vi "Get name from label.vi"(8 "error in (no error)":errorcluster, 10 "Selected label":string, 11 "UI JSON read cluster":T1) -> (0 "error out":errorcluster, 3 "Diagnostic name":string)   [LabVIEW 2019, in "ZenGage v3.0 UI.lvclass"]
uses:
  ZenGage v3.0 UI.lvclass
  Type Definitions/JSON Read/UI JSON read cluster.ctl
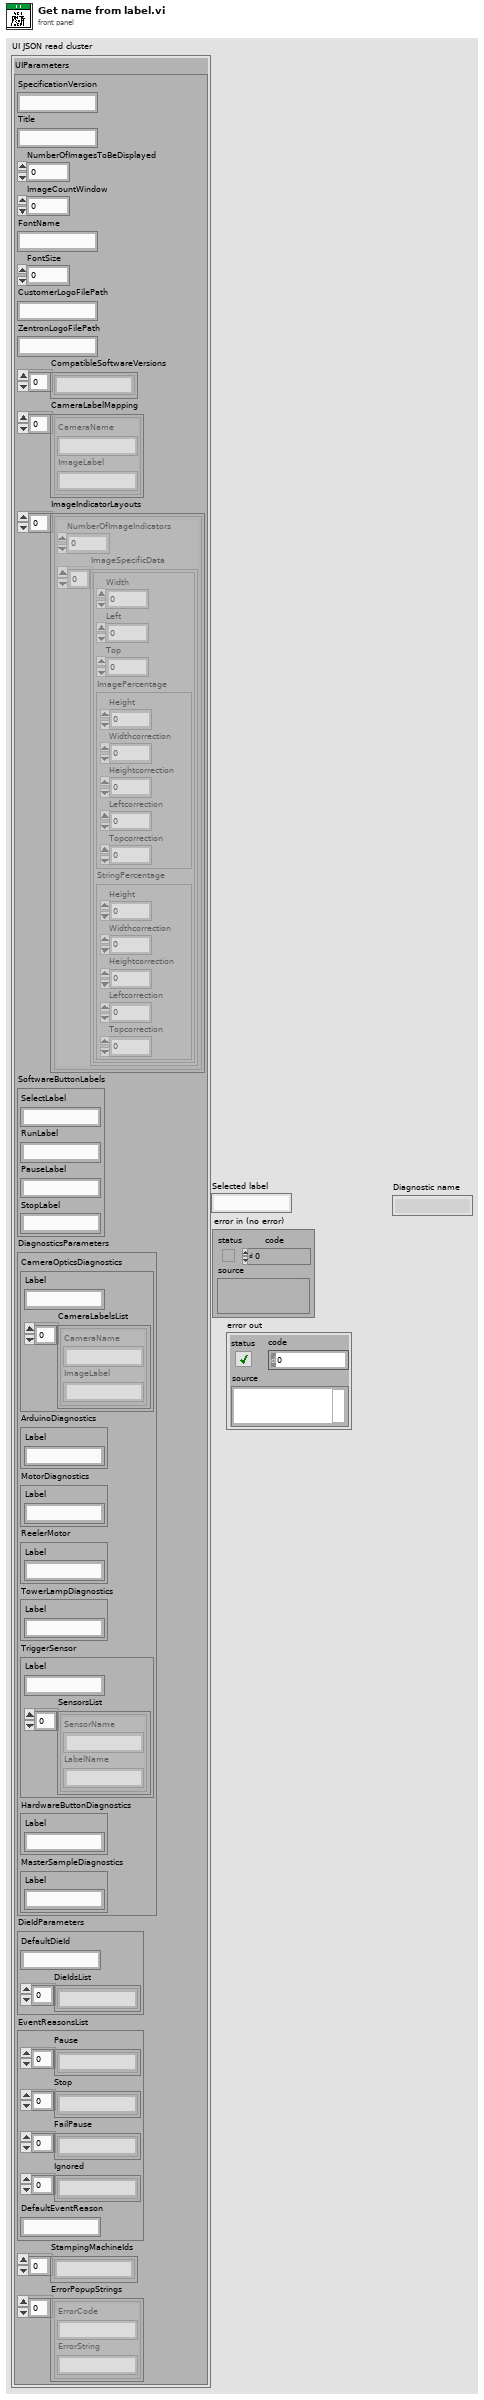
[diagram p1: front panel]
types:
  T1 = typedef "ZenGage v3.0 UI.lvclass/UI JSON read cluster.ctl" = cluster{"UIParameters":cluster{"SpecificationVersion":string, "Title":string, "NumberOfImagesToBeDisplayed":dbl, "ImageCountWindow":dbl, "FontName":string, "FontSize":dbl, "CustomerLogoFilePath":string, "ZentronLogoFilePath":string, "CompatibleSoftwareVersions":string[], "CameraLabelMapping":cluster{"CameraName":string, "ImageLabel":string}[], "ImageIndicatorLayouts":cluster{"NumberOfImageIndicators":dbl, "ImageSpecificData":cluster{"Width":dbl, "Left":dbl, "Top":dbl, "ImagePercentage":cluster{"Height":dbl, "Widthcorrection":i64, "Heightcorrection":i64, "Leftcorrection":dbl, "Topcorrection":dbl}, "StringPercentage":cluster{"Height":dbl, "Widthcorrection":i64, "Heightcorrection":dbl, "Leftcorrection":dbl, "Topcorrection":dbl}}[]}[], "SoftwareButtonLabels":cluster{"SelectLabel":string, "RunLabel":string, "PauseLabel":string, "StopLabel":string}, "DiagnosticsParameters":cluster{"CameraOpticsDiagnostics":cluster{"Label":string, "CameraLabelsList":cluster{"CameraName":string, "ImageLabel":string}[]}, "ArduinoDiagnostics":cluster{"Label":string}, "MotorDiagnostics":cluster{"Label":string}, "ReelerMotor":cluster{"Label":string}, "TowerLampDiagnostics":cluster{"Label":string}, "TriggerSensor":cluster{"Label":string, "SensorsList":cluster{"SensorName":string, "LabelName":string}[]}, "HardwareButtonDiagnostics":cluster{"Label":string}, "MasterSampleDiagnostics":cluster{"Label":string}}, "DieIdParameters":cluster{"DefaultDieId":string, "DieIdsList":string[]}, "EventReasonsList":cluster{"Pause":string[], "Stop":string[], "FailPause":string[], "Ignored":string[], "DefaultEventReason":string}, "StampingMachineIds":string[], "ErrorPopupStrings":cluster{"ErrorCode":string, "ErrorString":string}[]}}
  T2 = cluster{"CameraOpticsDiagnostics":cluster{"Label":string, "CameraLabelsList":cluster{"CameraName":string, "ImageLabel":string}[]}, "ArduinoDiagnostics":cluster{"Label":string}, "MotorDiagnostics":cluster{"Label":string}, "ReelerMotor":cluster{"Label":string}, "TowerLampDiagnostics":cluster{"Label":string}, "TriggerSensor":cluster{"Label":string, "SensorsList":cluster{"SensorName":string, "LabelName":string}[]}, "HardwareButtonDiagnostics":cluster{"Label":string}, "MasterSampleDiagnostics":cluster{"Label":string}}
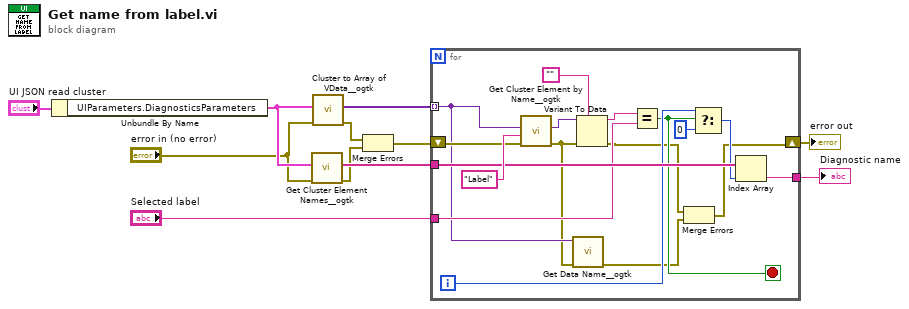
[diagram p0: block diagram]
diagram:
  n1 = Unbundle By Name("UI JSON read cluster") -> ("UIParameters.DiagnosticsParameters"=w10:T2)
  n2 = call <userlib>:"Get Cluster Element Names__ogtk.vi"("error in (no error)"="error in (no error)", "Cluster"=w10) -> ("error out"=w3:errorcluster, "Element Names"=w7:string[])  [unwired: 8 in]
  n3 = call <userlib>:"Cluster to Array of VData__ogtk.vi"("error in (no error)"="error in (no error)", "Cluster"=w10) -> ("error out"=w4:errorcluster, "Array of VData"=w9:variant[])  [unwired: 8 in]
  n4 = Merge Errors(w4, w3) -> (w2:errorcluster)
  n5 = for {
    tunnel: w9 -> [w16] mode=indexing
    tunnel: "Selected label" -> [w23]
    tunnel: w7 -> [w25]
    tunnel: [w19] -> w6
    shift-right: [w12] -> w1
    shift-left: w2 -> [w18]
    i -> [w22]
    stop <- w17 stop-if-true
    n6 = call <userlib>:"Get Cluster Element by Name__ogtk.vi"("error in (no error)"=w18, "Element Name"="Label", "Cluster"=w16) -> ("error out"=w15:errorcluster, "VElement"=w27:variant)  [unwired: 6 in, 1 out]
    n7 = call <userlib>:"Get Data Name__ogtk.vi"("error in (no error)"=w15, "Data"=w16) -> ("error out"=w14:errorcluster)  [unwired: 7 in, 2 out]
    n8 = Variant To Data(error in=w15, type="", Variant=w27) -> (data=w24:string, error out=w13:errorcluster)
    n9 = Equal?(x=w24, y=w23) -> (x = y?=w17:bool)
    n10 = Merge Errors(w13, w14) -> (w12:errorcluster)
    n11 = Select(t=w22, s=w17, f=0) -> (s? t:f=w20:i32)
    n12 = Index Array(array=w25, index=w20) -> (element=w19:string)
  }
  "Diagnostic name" <- w6
  "error out" <- w1
